vi "VMI_Image_type_settings_array.vi"(0 "Total Acquires":i32=1 caption="How many complete Acquires", 4 "Collection Information":T1[](array[typedef])) -> (1 "To Collect":i32, 6 "Image types Bool":bool[](array[boolean]), 7 "Number of Loops":i32)   [LabVIEW 2020]
uses:
  Type defs/FileAcq_v1_Ctrl.ctl
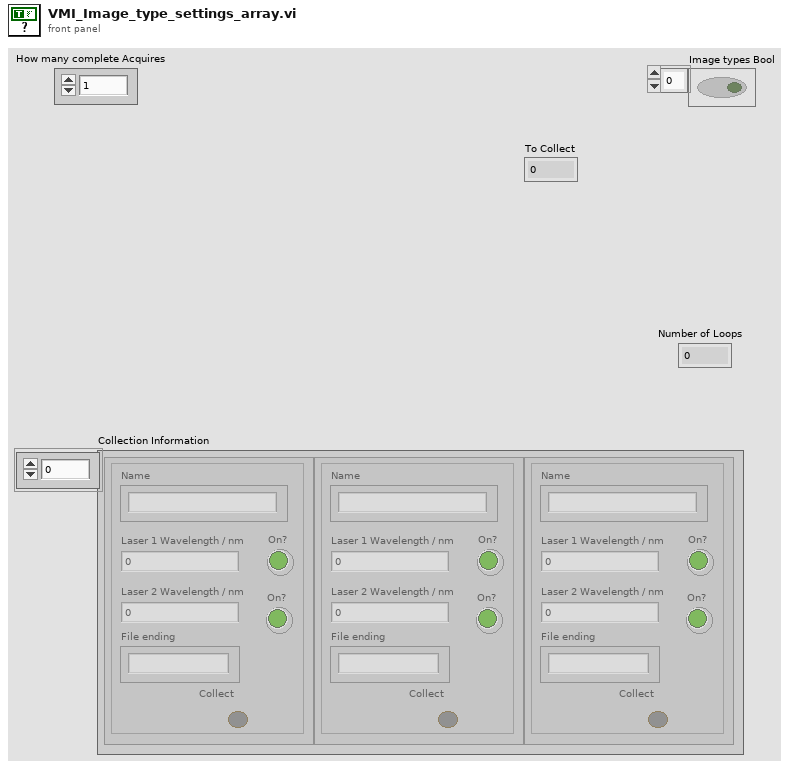
[diagram p1: front panel]
types:
  T1 = typedef "FileAcq_v1_Ctrl.ctl" = cluster{"Type":string, "LaserWave1":dbl, "Shutter1":bool, "LaserWave2":dbl, "Shutter2":bool, "FileEnd":string, "Collect":bool}
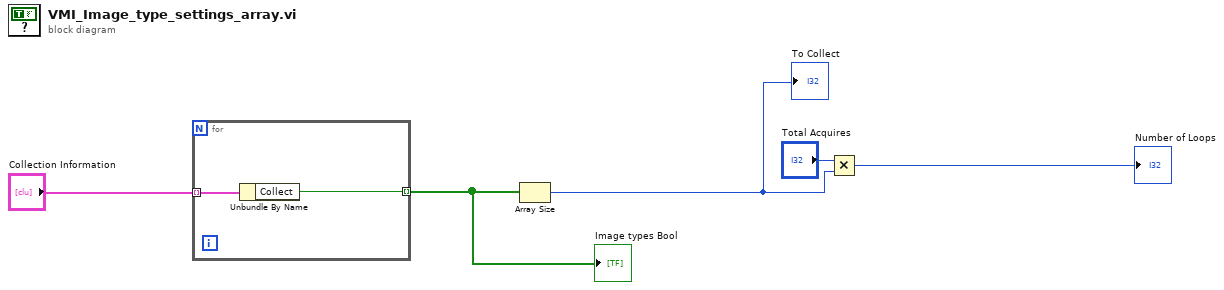
[diagram p0: block diagram]
diagram:
  n1 = for {
    tunnel: "Collection Information" -> [w7] mode=indexing
    tunnel: [w6] -> w1 mode=indexing
    n2 = Unbundle By Name(w7) -> ("Collect"=w6:bool)
  }
  "Image types Bool" <- w1
  n3 = Array Size(array=w1) -> (size(s)=w2:i32)
  "To Collect" <- w2
  n4 = Multiply(x="Total Acquires", y=w2) -> (x*y=→"Number of Loops":i32)
